vi "1D Scan.vi"(7 "Dwell Time (ms)":i32=10, 8 "Num Steps":i32, 9 "Step":dbl, 10 "Min":dbl, 11 "Channel":tag) -> (3 "Counts":i32[](array[numeric]))   [LabVIEW 2012]
uses:
  <vilib>/DAQmx/read.llb/DAQmx Read (Counter U32 1Chan 1Samp).vi
  <vilib>/DAQmx/write.llb/DAQmx Write (Analog DBL 1Chan 1Samp).vi
  <vilib>/DAQmx/create/channels.llb/DAQmx Create Channel (AO-Voltage-Basic).vi
  Channels.vi
  <vilib>/DAQmx/create/channels.llb/DAQmx Create Channel (CI-Count Edges).vi
  Global Vars.vi
  <vilib>/DAQmx/miscellaneous.llb/DAQmx Fill In Error Info.vi
panel:
  in  "Abort":bool
  out "AO Voltage":dbl
  out "Total Count":u32
  out "Current Count":i32
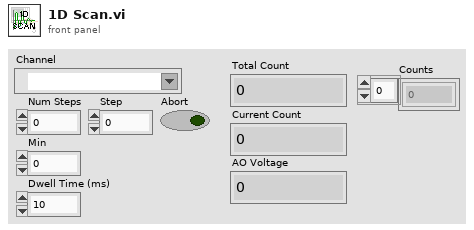
[diagram p1: front panel]
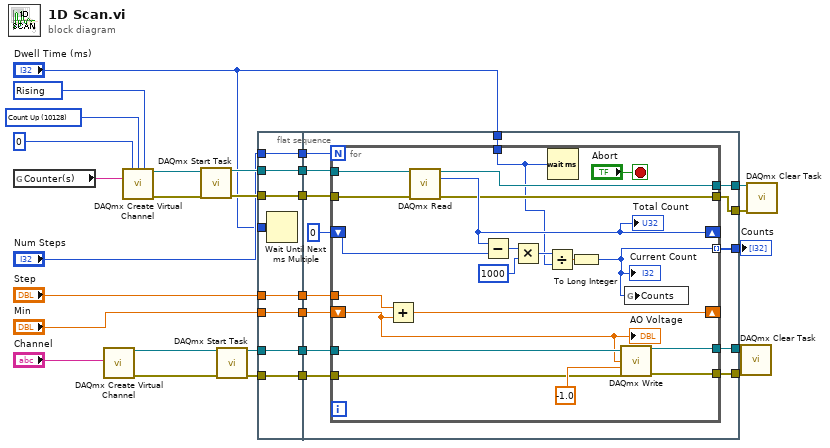
[diagram p0: block diagram]
diagram:
  w22 = 10280 items=["Rising"=10280, "Falling"=10171] ("Edge")
  w23 = 10128 items=["Count Up"=10128, "Count Down"=10124, "Externally Controlled"=10326] ("Count Direction")
  n1 = global read "Channels.vi" "Counter(s)"() -> (w21:tag)
  n2 = call-poly <vilib>:"DAQmx Create Virtual Channel.vi"("physical channels"="Channel") -> ("task out"=w28:refnum<k21>, "error out"=w27:errorcluster)  [unwired: 13 in]
  n3 = call-poly <vilib>:"DAQmx Create Virtual Channel.vi"("initial count"=u32 0 ("Initial Count"), "count direction"=w23, "edge"=w22, "counter"=w21) -> ("task out"=w20:refnum<k21>, "error out"=w18:errorcluster)  [unwired: 10 in]
  n4 = call <vilib>:"DAQmx Start Task.vi"("task/channels in"=w20, "error in"=w18) -> ("task out"=w19:refnum<k21>, "error out"=w17:errorcluster)  [unwired: 12 in]
  n5 = call <vilib>:"DAQmx Start Task.vi"("task/channels in"=w28, "error in"=w27) -> ("task out"=w26:refnum<k21>, "error out"=w25:errorcluster)  [unwired: 12 in]
  n6 = flat-sequence {
    tunnel: "Min" -> [w31]
    tunnel: "Step" -> [w32]
    tunnel: "Num Steps" -> [w33]
    tunnel: w17 -> [w34]
    tunnel: w19 -> [w35]
    tunnel: w25 -> [w36]
    tunnel: w26 -> [w37]
    tunnel: [w37] -> w8
    tunnel: [w36] -> w7
    tunnel: [w35] -> w6
    tunnel: [w34] -> w5
    tunnel: [w33] -> w4
    tunnel: [w32] -> w3
    tunnel: [w31] -> w2
    tunnel: "Dwell Time (ms)" -> [w30]
    tunnel: [w43] -> w13
    tunnel: "Dwell Time (ms)" -> [w42]
    tunnel: [w41] -> w12
    tunnel: [w40] -> w11
    tunnel: [w39] -> w10
    tunnel: [w38] -> w9
    tunnel: w8 -> [w51]
    tunnel: w7 -> [w50]
    tunnel: w6 -> [w49]
    tunnel: w5 -> [w48]
    tunnel: w4 -> [w46]
    tunnel: w3 -> [w45]
    tunnel: w2 -> [w44]
    frame #0 {
      n7 = Wait Until Next ms Multiple(millisecond multiple=w30) -> ()  [unwired: 1 out]
    }
    frame #1 {
      n8 = for {
        N: w46 -> [_]
        shift-right: [w72] -> _
        shift-left: w44 -> [w62]
        tunnel: [w70] -> w41
        tunnel: [w69] -> w40
        shift-right: [w68] -> _
        shift-left: 0 -> [w67]
        tunnel: [w52] -> w43 mode=indexing
        tunnel: w51 -> [w66]
        tunnel: w50 -> [w65]
        tunnel: w49 -> [w64]
        tunnel: w48 -> [w63]
        tunnel: w45 -> [w61]
        tunnel: w42 -> [w54]
        tunnel: [w59] -> w39
        tunnel: [w58] -> w38
        stop <- "Abort" stop-if-true
        n9 = Add(x=w61, y=w62) -> (x+y=w72:dbl)
        n10 = call-poly <vilib>:"DAQmx Read.vi"("task/channels in"=w64, "error in"=w63) -> ("task out"=w59:refnum<k21>, "data"=w68:u32, "error out"=w58:errorcluster)  [unwired: 11 in]
        "Total Count" <- w68
        n11 = Subtract(x=w68, y=w67) -> (x-y=w57:u32)
        n12 = Multiply(x=w57, y=1000) -> (x*y=w55:u32)
        n13 = Divide(x=w55, y=w54) -> (x/y=w53:dbl)
        n14 = Wait (ms)(milliseconds to wait=w54) -> ()  [unwired: 1 out]
        n15 = To Long Integer(number=w53) -> (32bit integer=w52:i32)
        "Current Count" <- w52
        n16 = call-poly <vilib>:"DAQmx Write.vi"("task/channels in"=w66, "data"=w62, "timeout"=-1.0, "error in"=w65) -> ("task out"=w70:refnum<k21>, "error out"=w69:errorcluster)  [unwired: 9 in, 1 out]
        n17 = global write "Global Vars.vi" "Counts"(w52) -> ()
        "AO Voltage" <- w62
      }
    }
  }
  n18 = call <vilib>:"DAQmx Clear Task.vi"("task in"=w12, "error in"=w11) -> ()  [unwired: 13 in, 1 out]
  n19 = call <vilib>:"DAQmx Clear Task.vi"("task in"=w10, "error in"=w9) -> ()  [unwired: 13 in, 1 out]
  "Counts" <- w13
